vi "test7-StateBroadcast_Queue.vi"(8 "error in (no error)":errorcluster, 11 "TestCase in":refnum<class "testcase-CSMGlobalLog.lvclass">) -> (0 "error out":errorcluster, 3 "TestCase out":refnum<class "testcase-CSMGlobalLog.lvclass">)   [LabVIEW 2017, in "testcase-CSMGlobalLog.lvclass"]
uses:
  testcase-CSMGlobalLog.lvclass
  testcase-CSMGlobalLog.lvclass/testcase-CSMGlobalLog.ctl
  1e8c9b29-fab4-4a33-a8e9-8470233780e8.vi
  a5f4639e-abb1-4dab-bc02-210f1612dc56.vi
  84c2dbf3-f342-470d-873d-89135090fc9c.vi
  <vilib>/addons/_JKI Toolkits/VI Tester/TestCase.llb/TestCase.lvclass
  src/user.lib/_NEVSTOP/Communicable State Machine(CSM)/Communicable State Machine.lvlib
  src/user.lib/_NEVSTOP/Communicable State Machine(CSM)/Utility/Periodic String Filter Setting.ctl
  C:/Program Files (x86)/National Instruments/LabVIEW 2017/vi.lib/addons/_JKI Toolkits/VI Tester/TestCase.llb/TestCase.lvclass
panel:
  out "String cache total":string
  out "LoopCount":i32
  out "String Cache Each Loop":string
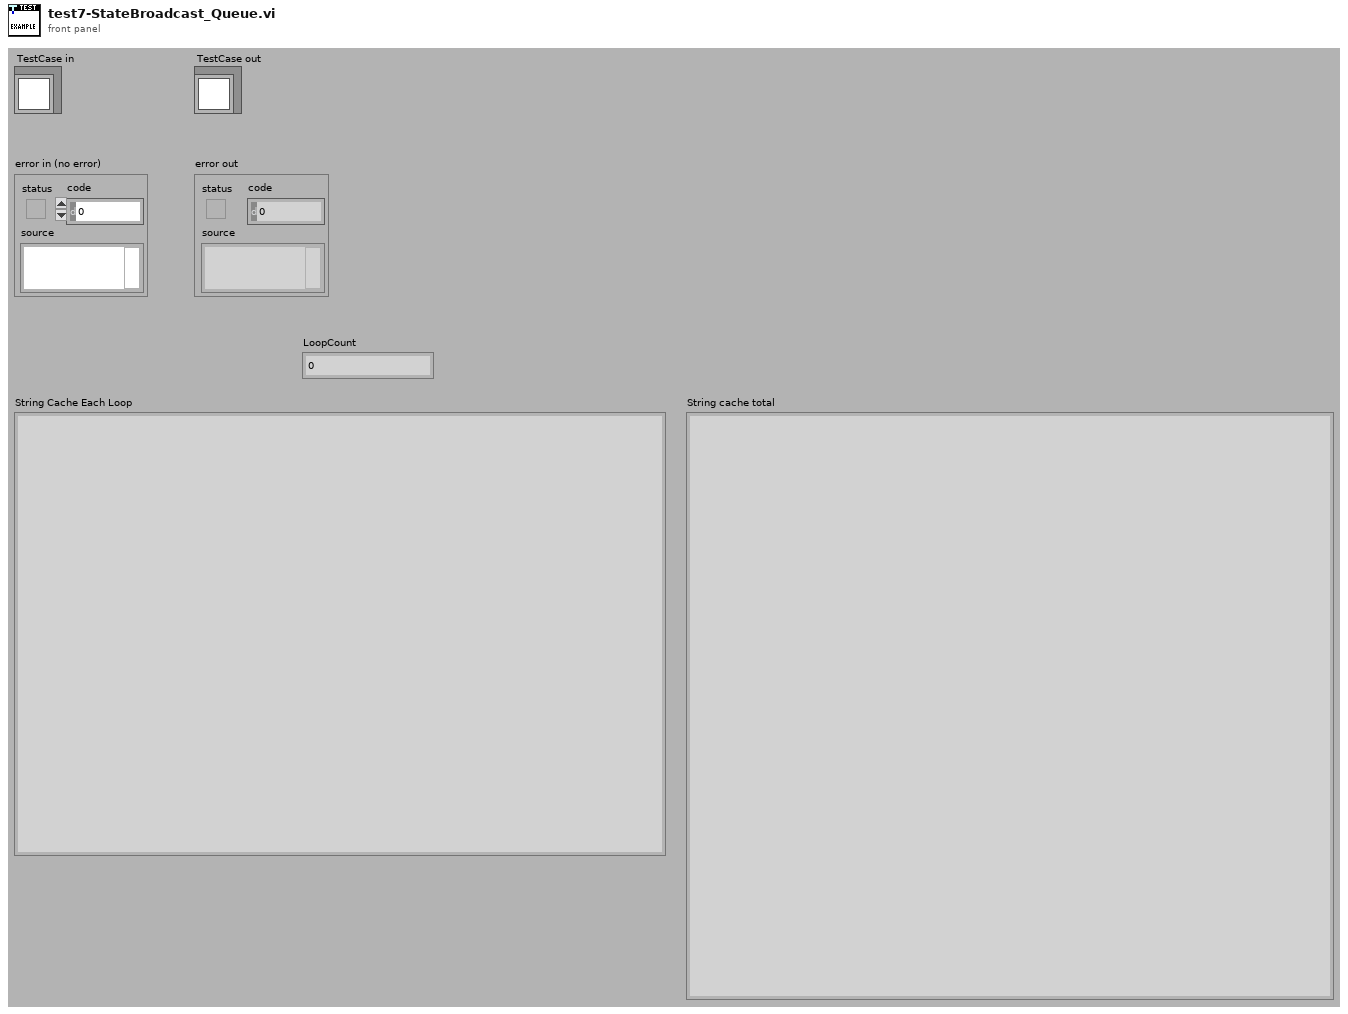
[diagram p1: front panel]
types:
  T1 = typedef "Communicable State Machine.lvlib/Periodic String Filter Setting.ctl" = cluster{"threashold(#/s)":dbl, "Check Peroid(s)":dbl}
  T2 = typedef "Communicable State Machine.lvlib/_CSM_GlobalLog_MSG.ctl" = cluster{"Name (\"\" to Use UUID)":string, "Current State":string, "Arguments":string, "Source Message":T3, "Source Module":string, "Complete(T)/Start(F)":bool, "LogType":T4, "Time Stamp":timestamp}
  T3 = typedef "Communicable State Machine.lvlib/_CSM_Response Source Message.ctl" = cluster{"‘State":string, "’Arguments":string, "’Error":errorcluster}
  T4 = typedef "Communicable State Machine.lvlib/_CSM_GlobalLog_MSG_TYPE.ctl" = enum16{"User Log", "State Change", "Status", "Interrupt", "Register", "Unregister", "Error Log", "Module Created", "Module Destroyed", "Async Message", "No-Rep Async Message", "Sync Message"}
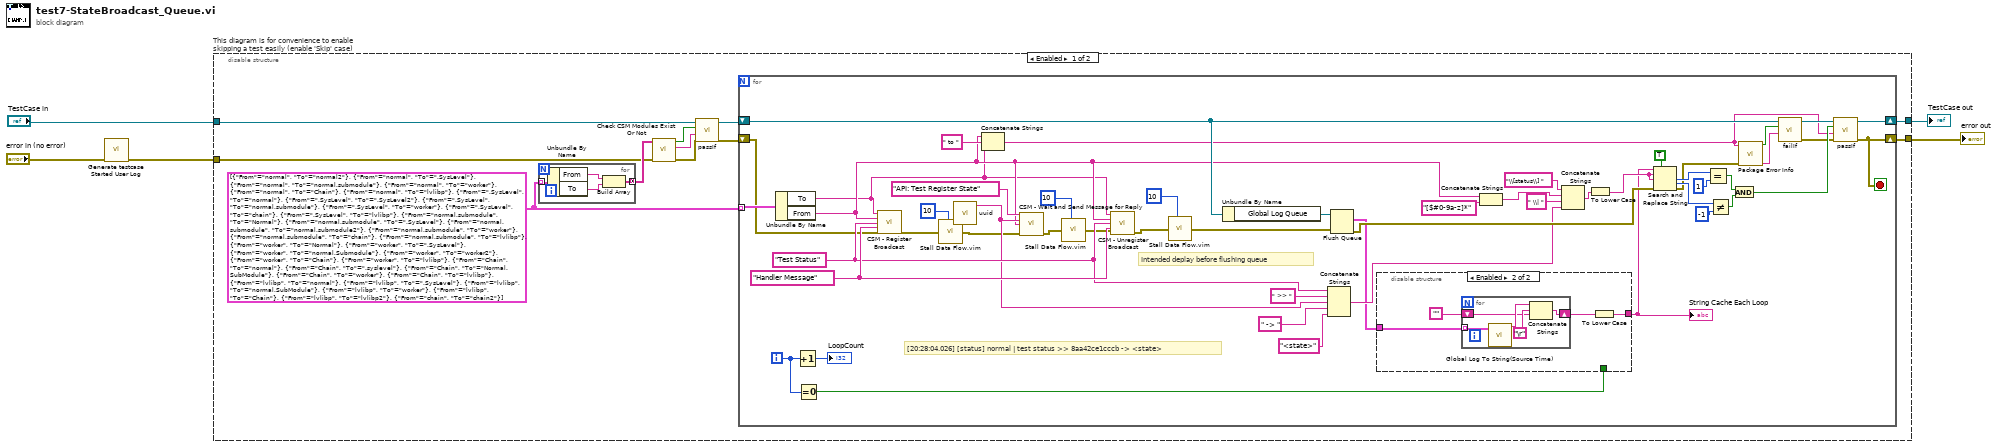
[diagram p0: block diagram]
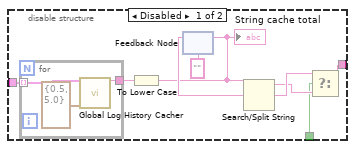
[diagram p2: hidden frame]
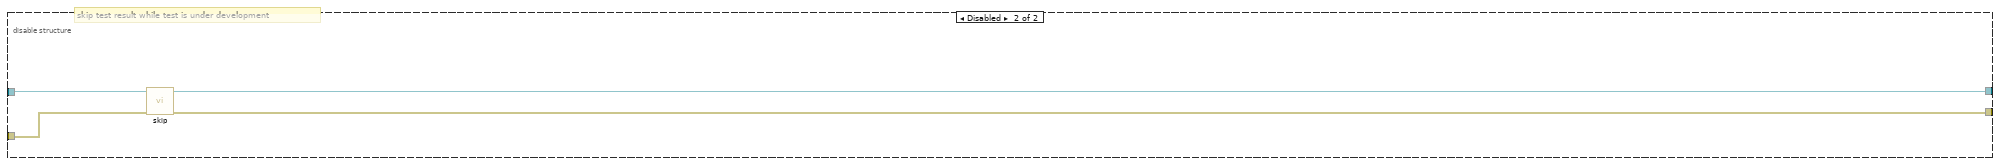
[diagram p3: hidden frame]
diagram:
  n1 = call "Generate testcase Started User Log.vi"("Error In"="error in (no error)") -> ("error out"=w1:errorcluster)  [unwired: 10 in]
  n2 = disable-structure "This diagram is for convenience to enable skipping a test easily (enable 'Skip' case)" shown="Enabled" {
    disable-tunnel: "TestCase in" -> [w9 w97]
    disable-tunnel: [w15 w95] -> w2
    disable-tunnel: [w16 w96] -> w4
    disable-tunnel: w1 -> [w6 w94]
    frame Enabled {
      w10 = cluster{"From":string, "To":string}[] [{"From"="normal", "To"="normal2"}, {"From"="normal", "To"=".SysLevel"}, {"From"="normal", "To"="normal.submodule"}, {"From"="normal", "To"="worker"}, {"From"="normal", "To"="Chain"}, {"From"="normal", "To"="lvlibp"}, {"From"=".SysLevel", "To"="normal"}, {"From"=".SysLevel", "To"=".SysLevel2"}, {"From"=".SysLevel", "To"="normal.submodule"}, {"From"=".SysLevel", "To"="worker"}, {"From"=".SysLevel", "To"="chain"}, {"From"=".SysLevel", "To"="lvlibp"}, {"From"="normal.submodule", "To"="Normal"}, {"From"="normal.submodule", "To"=".SysLevel"}, {"From"="normal.submodule", "To"="normal.submodule2"}, {"From"="normal.submodule", "To"="worker"}, {"From"="normal.submodule", "To"="chain"}, {"From"="normal.submodule", "To"="lvlibp"}, {"From"="worker", "To"="Normal"}, {"From"="worker", "To"=".SysLevel"}, {"From"="worker", "To"="normal.Submodule"}, {"From"="worker", "To"="worker2"}, {"From"="worker", "To"="Chain"}, {"From"="worker", "To"="lvlibp"}, {"From"="Chain", "To"="normal"}, {"From"="Chain", "To"=".syslevel"}, {"From"="Chain", "To"="Normal.SubModule"}, {"From"="Chain", "To"="worker"}, {"From"="Chain", "To"="lvlibp"}, {"From"="lvlibp", "To"="normal"}, {"From"="lvlibp", "To"=".SysLevel"}, {"From"="lvlibp", "To"="normal.SubModule"}, {"From"="lvlibp", "To"="worker"}, {"From"="lvlibp", "To"="Chain"}, {"From"="lvlibp", "To"="lvlibp2"}, {"From"="chain", "To"="chain2"}]
      n3 = for {
        tunnel: w10 -> [w20] mode=indexing
        tunnel: [w17] -> w13 mode=concatenating
        n4 = Unbundle By Name(w20) -> ("From"=w19:string, "To"=w18:string)
        n5 = Build Array(w19, w18) -> (w17:string[])
      }
      n6 = call "Check CSM Modules Exist Or Not.vi"("error in"=w6, "CSM names in"=w13) -> ("error out"=w11:errorcluster, "Debug string"=w12:string, "All Modules Exist?"=w14:bool)  [unwired: 7 in]
      n7 = call-dynamic "passIf.vi"("error in (no error)"=w11, "message (\"\")"=w12, "pass"=w14, "TestCase in"=w9) -> ("error out"=w7:errorcluster, "TestCase out"=w8:refnum<class "testcase-CSMGlobalLog.lvclass">)  [unwired: 6 in]
      n8 = for {
        tunnel: w10 -> [w60] mode=indexing
        shift-right: [w46] -> w16
        shift-left: w7 -> [w37]
        shift-right: [w72] -> w15
        shift-left: w8 -> [w34]
        i -> [w39]
        stop <- w46 stop-if-true
        w59 = "Handler Message" ("API (If \"\", Same as Trigger)")
        w54 = "Test Status" ("Trigger")
        # "[20:28:04.026] [status] normal | test status >> 8aa42ce1cccb -> <state>"
        # "Intended deplay before flushing queue"
        n9 = Unbundle By Name(w60) -> ("To"=w28:string, "From"=w29:string)
        n10 = Increment(x=w39) -> (x+1=→"LoopCount":i32)
        n11 = Equal To 0?(x=w39) -> (x = 0?=w38:bool)
        n12 = call "CSM - Register Broadcast.vi"("CSM Name(Empty for Broadcast Event)"=w28, "Source CSM Name (* as Default)"=w29, "Trigger"=w54, "API (If \"\", Same as Trigger)"=w59, "Error In"=w37) -> ("error out"=w22:errorcluster)  [unwired: 9 in, 1 out]
        n13 = call "Stall Data Flow.vim"("value in"=w22, "milliseconds to wait"=u32 10) -> ("value out"=w21:errorcluster)  [unwired: 1 out]
        n14 = call "uuid.vi"() -> ("UUID"=w52:string)  [unwired: 11 in]
        n15 = Concatenate Strings(w29, " to " ("string"), w28) -> (w27:string)
        n16 = call "CSM - Wait and Send Message for Reply.vi"("State"="API: Test Register State", "Arguments (\"\")"=w52, "Target Module"=w29, "Error In (No Error)"=w21) -> ("error out"=w25:errorcluster)  [unwired: 8 in, 3 out]
        n17 = call "Stall Data Flow.vim"("value in"=w25, "milliseconds to wait"=u32 10) -> ("value out"=w24:errorcluster)  [unwired: 1 out]
        n18 = call "CSM - Unregister Broadcast.vi"("CSM Name(Empty for Broadcast Event)"=w28, "Source CSM Name (* as Default)"=w29, "Trigger"=w54, "API (\"*\" as Default)"=w59, "Error In"=w24) -> ("error out"=w44:errorcluster)  [unwired: 9 in, 1 out]
        n19 = call "Stall Data Flow.vim"("value in"=w44, "milliseconds to wait"=u32 10) -> ("value out"=w43:errorcluster)  [unwired: 1 out]
        n20 = Unbundle By Name(w34) -> ("Global Log Queue"=w71:refnum<queue>)
        n21 = Concatenate Strings(w54, " >> " ("string"), w52, " -> " ("string"), "<state>" ("search string")) -> (w50:string)
        n22 = Flush Queue(queue=w71, error in (no error)=w43) -> (remaining elements=w40:T2[], error out=w62:errorcluster)  [unwired: 1 out]
        n23 = disable-structure shown="Enabled" {
          disable-tunnel: [w75 w85] -> w41
          disable-tunnel: w38 -> [w74 _]
          disable-tunnel: w40 -> [w73 w87]
          frame Disabled {
            n24 = for {
              tunnel: w73 -> [w84] mode=indexing
              tunnel: [w83] -> w81
              n25 = call "Global Log History Cacher.vi"("Global Log Data"=w84, "Settings"=T1 {"threashold(#/s)"=0.5, "Check Peroid(s)"=5.0}) -> ("String Cache"=w83:string)  [unwired: 13 in]
            }
            n26 = To Lower Case(string=w81) -> (all lower case string=w76:string)
            "String cache total" <- w76
            n27 = feedback #1("") -> (w80:string)
            n28 = feedback-in #1(w76) -> ()
            n29 = Search/Split String(string=w76, search string/char (-)=w80) -> (substring before match=w77:string, match + rest of string=w78:string)  [unwired: 1 in, 1 out]
            n30 = Select(t=w78, s=w74, f=w77) -> (s? t:f=w75:string)
          }
          frame Enabled {
            n31 = for {
              tunnel: w87 -> [w93] mode=indexing
              shift-right: [w89] -> w86
              shift-left: "" -> [w90]
              n32 = call "Global Log To String(Source Time).vi"("Log"=w93) -> ("Log String"=w92:string)  [unwired: 9 in]
              n33 = Concatenate Strings(w92, "\r", w90) -> (w89:string)
            }
            n34 = To Lower Case(string=w86) -> (all lower case string=w85:string)
          }
        }
        "String Cache Each Loop" <- w41
        n35 = Concatenate Strings(w29, "[$#0-9a-z]*" ("string")) -> (w47:string)
        n36 = Concatenate Strings("\\[status\\] " ("regular expression"), w47, " \\| " ("string"), w50) -> (w56:string)
        n37 = To Lower Case(string=w56) -> (all lower case string=w68:string)
        n38 = Search and Replace String(replace all?=TRUE ("replace all? (F)"), input string=w41, search string=w68, replace string=w68, error in=w62) -> (number of replacements=w67:i32, offset past replacement=w66:i32, error out=w31:errorcluster)  [unwired: 3 in, 1 out]
        n39 = Equal?(x=w67, y=1) -> (x = y?=w64:bool)
        n40 = Not Equal?(x=w66, y=-1) -> (x != y?=w63:bool)
        n41 = And(x=w64, y=w63) -> (x .and. y?=w45:bool)
        n42 = call "Package Error Info.vi"("error in"=w31, "String in"=w27) -> ("packed error info out"=w35:string, "error status"=w36:bool)  [unwired: 8 in]
        n43 = call-dynamic "failIf.vi"("message (\"\")"=w35, "fail"=w36, "TestCase in"=w34) -> ("error out"=w32:errorcluster, "TestCase out"=w33:refnum<class "testcase-CSMGlobalLog.lvclass">)  [unwired: 7 in]
        n44 = call-dynamic "passIf.vi"("error in (no error)"=w32, "message (\"\")"=w27, "pass"=w45, "TestCase in"=w33) -> ("error out"=w46:errorcluster, "TestCase out"=w72:refnum<class "testcase-CSMGlobalLog.lvclass">)  [unwired: 6 in]
      }
    }
    frame Disabled {
      # "skip test result while test is under development"
      n45 = call <vilib>:"skip.vi"("error in (no error)"=w94, "TestCase in"=w97) -> ("error out"=w96:errorcluster, "TestCase out"=w95:refnum<class "testcase-CSMGlobalLog.lvclass">)  [unwired: 8 in]
    }
  }
  "error out" <- w4
  "TestCase out" <- w2
